vi "CSTK_Enum_Creator_Core_Create.vi"(6 "标签名":string, 8 "错误输入（无错误）":errorcluster, 9 "项名":string, 10 "样式":u32(ring)=3062 items=["枚举（经典）"=3023, "枚举（系统）"=3062, "枚举（新式）"=21605]) -> (0 "错误输出":errorcluster)   [LabVIEW 2015, in "CSTK_Enum Creator.lvlib"]
uses:
  CSTK_Enum Creator.lvlib
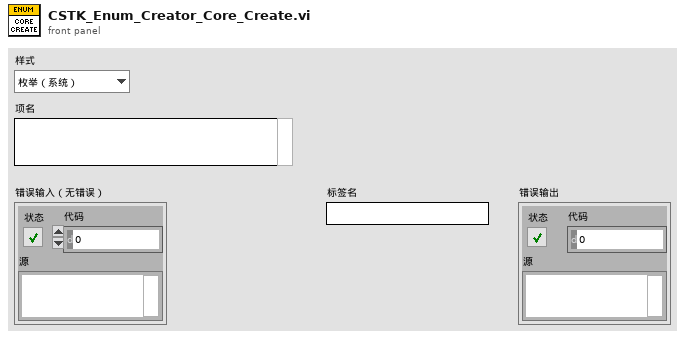
[diagram p1: front panel]
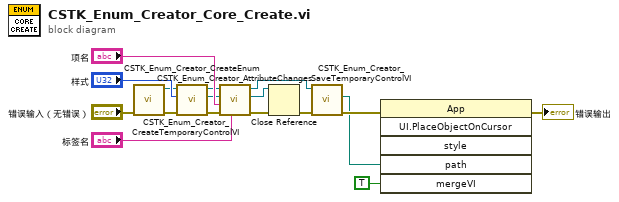
[diagram p0: block diagram]
diagram:
  n1 = call "CSTK_Enum_Creator_CreateTemporaryControlVI.vi"("错误输入（无错误）"="错误输入（无错误）") -> ("错误输出"=w15:errorcluster, "VI输出"=w11:refnum<vi>)  [unwired: 9 in]
  n2 = call "CSTK_Enum_Creator_CreateEnum.vi"("错误输入（无错误）"=w15, "样式"="样式", "VI输入"=w11) -> ("错误输出"=w17:errorcluster, "Enum输出"=w10:refnum<vi>, "VI输出"=w9:refnum<vi>)  [unwired: 6 in]
  n3 = call "CSTK_Enum_Creator_AttributeChanges.vi"("标签名"="标签名", "错误输入（无错误）"=w17, "项名"="项名", "Enum输入"=w10, "VI输入"=w9) -> ("错误输出"=w2:errorcluster, "Enum输出"=w3:refnum<vi>, "VI输出"=w7:refnum<vi>)  [unwired: 4 in]
  n4 = Close Reference(reference=w3, error in (no error)=w2) -> (error out=w1:errorcluster)
  n5 = call "CSTK_Enum_Creator_SaveTemporaryControlVI.vi"("错误输入（无错误）"=w1, "VI输入"=w7) -> ("错误输出"=w14:errorcluster, "存储路径输出"=w6:path)  [unwired: 8 in]
  n6 = invoke class="App" method="UI.PlaceObjectOnCursor"(error in=w14, "path"=w6, "mergeVI"=TRUE ("合并VI")) -> (error out=→"错误输出":errorcluster)  [unwired: 3 in, 5 out]
